vi "UI Update table row color.vi"(9 "Data":string[](array[string]), 10 "index of element":i32, 11 "Table in":refnum<vi>) -> (2 "Alarm":bool)   [LabVIEW 2020]
uses:
  <vilib>/Utility/miscctls.llb/LVRowAndColumnTypeDef.ctl
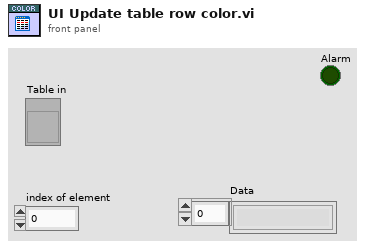
[diagram p1: front panel]
types:
  T1 = typedef "LVRowAndColumnTypeDef.ctl" = cluster{"Row":i32, "Column":i32}
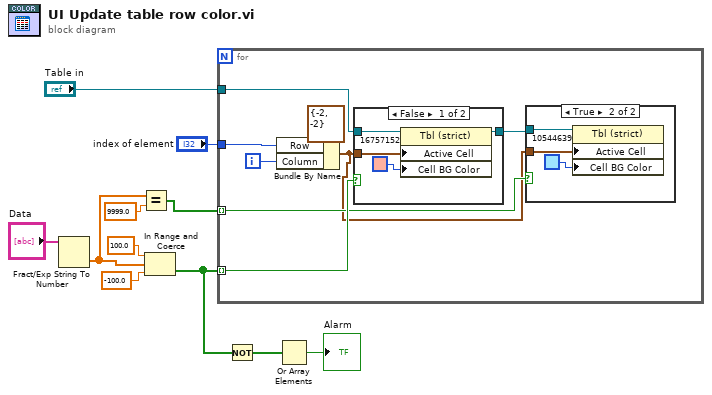
[diagram p0: block diagram]
diagram:
  n1 = Fract/Exp String To Number(string="Data") -> (number=w3:dbl[])  [unwired: 3 in, 1 out]
  n2 = Equal?(x=w3, y=9999.0) -> (x = y?=w1:bool[])
  n3 = In Range and Coerce(upper limit=100.0, x=w3, lower limit=-100.0) -> (In Range?=w6:bool[])  [unwired: 1 out]
  n4 = for {
    tunnel: "index of element" -> [w19]
    tunnel: "Table in" -> [w17]
    tunnel: w6 -> [w16] mode=indexing
    tunnel: w1 -> [w14] mode=indexing
    i -> [w15]
    n5 = Bundle By Name(cluster=T1 {"Row"=-2, "Column"=-2} ("Active Cell:Active Cell"), "Row"=w19, "Column"=w15) -> (w12:T1)
    n6 = case shown="False" w16 {
      tunnel: w12 -> [w26 _]
      tunnel: w17 -> [w25 w27]
      tunnel: [w23 w27] -> w13
      frame False {
        n7 = property class="Tbl (strict)"(reference=w25, "Active Cell"=w26, "Cell BG Color"=u32 16757152) -> (reference out=w23:refnum<vi>)  [unwired: 1 in, 1 out]
      }
      frame True {
      }
    }
    n8 = case shown="True" w14 {
      tunnel: w12 -> [_ w22]
      tunnel: w13 -> [_ w21]
      frame False {
      }
      frame True {
        n9 = property class="Tbl (strict)"(reference=w21, "Active Cell"=w22, "Cell BG Color"=u32 10544639) -> ()  [unwired: 1 in, 2 out]
      }
    }
  }
  n10 = Not(x=w6) -> (.not. x?=w4:bool[])
  n11 = Or Array Elements(Boolean array=w4) -> (logical OR=→"Alarm":bool)
